vi "_to_comparable_map.vi"(11 "httpHeaders in":refnum<class "httpHeaders.lvclass">) -> (3 "comparable headers":cluster{"header":string, "value":string}[](array[cluster]))   [LabVIEW 2020, in "httpClient.lvlib" / "httpHeaders.lvclass"]
uses:
  httpHeaders.lvclass
  httpHeaders.lvclass/httpHeaders.ctl
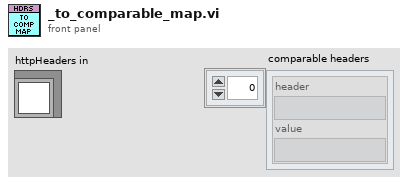
[diagram p1: front panel]
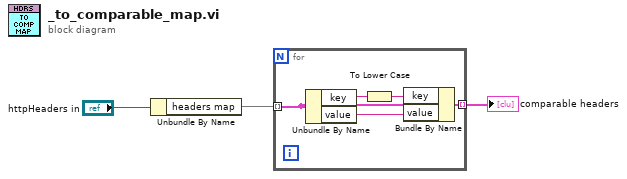
[diagram p0: block diagram]
diagram:
  n1 = Unbundle By Name("httpHeaders in") -> ("headers map"=w2:map{string, string})
  n2 = for {
    tunnel: w2 -> [w7] mode=indexing
    tunnel: [w4] -> w1 mode=indexing
    n3 = Unbundle By Name(w7) -> ("key"=w8:string, "value"=w5:string)
    n4 = To Lower Case(string=w8) -> (all lower case string=w6:string)
    n5 = Bundle By Name(cluster=w7, "key"=w6, "value"=w5) -> (w4:cluster{"key":string, "value":string})
  }
  "comparable headers" <- w1
